vi "数字或字母的GB2312编码山推.vi"(10 "正则表达式":string, 11 "显示字符输入":string) -> (3 "显示字符输出":string)   [LabVIEW 2016]
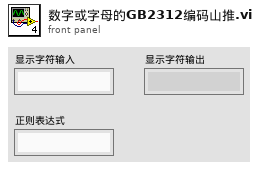
[diagram p1: front panel]
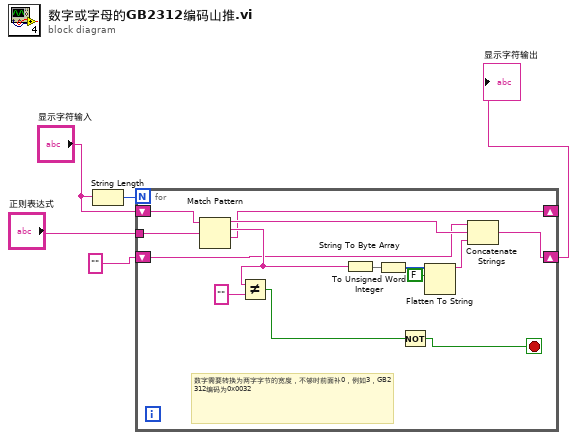
[diagram p0: block diagram]
diagram:
  n1 = String Length(string="显示字符输入") -> (length=w2:i32)
  n2 = for {
    N: w2 -> [_]
    shift-right: [w11] -> _
    shift-left: "显示字符输入" -> [w19]
    shift-right: [w8] -> w4
    shift-left: "" ("显示字符") -> [w7]
    tunnel: "正则表达式" -> [w6]
    stop <- w10 stop-if-true
    # "数字需要转换为两字字节的宽度，不够时前面补0，例如3，GB2312编码为0x0032"
    n3 = Match Pattern(string=w19, regular expression=w6) -> (before substring=w14:string, match substring=w13:string, after substring=w11:string)  [unwired: 1 in, 1 out]
    n4 = Not Equal?(x=w13, y="") -> (x != y?=w9:bool)
    n5 = String To Byte Array(string=w13) -> (unsigned byte array=w18:u8[])
    n6 = To Unsigned Word Integer(number=w18) -> (unsigned 16bit integer=w17:u16[])
    n7 = Not(x=w9) -> (.not. x?=w10:bool)
    n8 = Flatten To String(anything=w17, prepend array or string size? (T)=FALSE ("预置数组或字符串大小？ (T)")) -> (data string=w15:string)  [unwired: 2 in, 2 out]
    n9 = Concatenate Strings(w7, w14, w15) -> (w8:string)
  }
  "显示字符输出" <- w4
